vi "Find Node By Name.vi"(0 "FSM.Graph":refnum<class "FSM.Graph.lvclass">, 7 "Name":string) -> (8 "Node":refnum<class "FSM.Node.lvclass">, 15 "index":i32)   [LabVIEW 2020, in "FSM.Graph.lvclass"]
uses:
  FSM.Graph.lvclass
  FSM.Node/FSM.Node.lvclass
  FSM.Graph.lvclass/FSM.Graph.ctl
  FSM.Node/FSM.Node.lvclass/FSM.Node.ctl
  FSM.Node/Read Name.vi
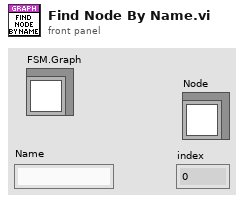
[diagram p1: front panel]
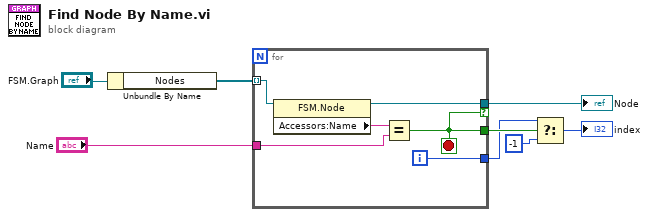
[diagram p0: block diagram]
diagram:
  n1 = Unbundle By Name("FSM.Graph") -> ("Nodes"=w7:refnum<class "FSM.Node.lvclass">[])
  n2 = for {
    tunnel: w7 -> [w14] mode=indexing
    tunnel: "Name" -> [w12]
    tunnel: [w11] -> w5 if=w9
    tunnel: [w10] -> w3
    tunnel: [w9] -> w4
    i -> [w10]
    stop <- w9 stop-if-true
    n3 = property class="FSM.Node"(reference=w14) -> (reference out=w11:refnum<class "FSM.Node.lvclass">, "Accessors:Name"=w13:string)  [unwired: 1 in, 1 out]
    n4 = Equal?(x=w13, y=w12) -> (x = y?=w9:bool)
  }
  "Node" <- w5
  n5 = Select(t=w3, s=w4, f=-1) -> (s? t:f=→"index":i32)
